vi "FTW-JSON-Object-SetElement-DBL.vi"(0 "JSON Object":refnum<data-value>, 5 "Key":string, 7 "Value":dbl, 11 "error in":errorcluster) -> (4 "JSON Object out":refnum<data-value>, 15 "error out":errorcluster)   [LabVIEW 2014]
uses:
  core/FTW-JSON-Core-Structure.ctl
  error/FTW-ERR-ThrowGenericError.vi
  error/FTW-ERR-ThrowError.vi
  error/FTW-ERR-NoErrorConstant.vi
  error/FTW-ERR-CallChain.vi
  string/FTW-STR-ReplaceWhitespace.vi
panel:
  # "Inputs"
  # "Outputs"
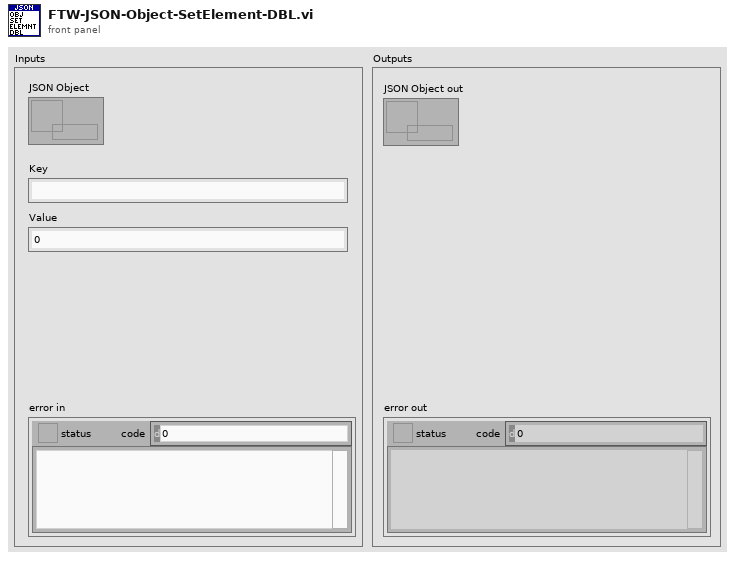
[diagram p1: front panel]
types:
  T1 = typedef "FTW-JSON-Core-Structure.ctl" = cluster{"JSON Object":i64, "Encoding Flags":i64, "Decoding Flags":i64}
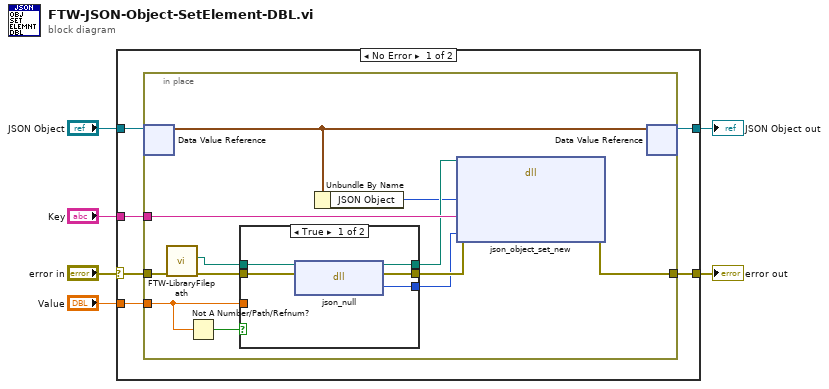
[diagram p0: block diagram]
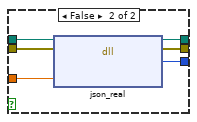
[diagram p2: hidden frame]
diagram:
  n1 = case shown="No Error" "error in" {
    selector: "error in" -> [w12 w37]
    tunnel: [w11 w37] -> w6
    tunnel: [w7 w36] -> w4
    tunnel: "JSON Object" -> [w8 w36]
    tunnel: "Key" -> [w10 _]
    tunnel: "Value" -> [w9 _]
    frame No Error {
      n2 = in-place {
        in-place-border: w12 -> [w24]
        in-place-border: [w23] -> w11
        in-place-border: w10 -> [w22]
        in-place-border: w9 -> [w16]
        n3 = in-place-dvr #1(w8) -> (w14:T1)  [unwired: 1 out]
        n4 = call "FTW-LibraryFilepath.vi"("error in"=w24) -> ("error out"=w19:errorcluster, "Library Filepath"=w21:path)  [unwired: 8 in, 1 out]
        n5 = Not A Number/Path/Refnum?(number/path/refnum=w16) -> (NaN/Path/Refnum?=w15:bool)
        n6 = case shown="True" w15 {
          tunnel: w21 -> [w29 w35]
          tunnel: [w28 w34] -> w20
          tunnel: w19 -> [w27 w33]
          tunnel: [w26 w32] -> w18
          tunnel: w16 -> [_ w31]
          tunnel: [w25 w30] -> w17
          frame True {
            n7 = dll-call lib="?" fn="json_null"(path in=w29, error in=w27) -> (path out=w28:path, error out=w26:errorcluster, "null Value"=w25:i64)  [unwired: 1 in]
          }
          frame False {
            n8 = dll-call lib="?" fn="json_real"(path in=w35, error in=w33, "Double Value"=w31) -> (path out=w34:path, error out=w32:errorcluster, "New Double Value"=w30:i64)  [unwired: 2 in]
          }
        }
        n9 = Unbundle By Name(w14) -> ("JSON Object"=w13:i64)
        n10 = dll-call lib="?" fn="json_object_set_new"(path in=w20, error in=w18, "JSON Object Pointer"=w13, "Key"=w22, "New JSON Object"=w17) -> (error out=w23:errorcluster)  [unwired: 5 in, 1 out]
        n11 = in-place-dvr #1(w14) -> (w7:refnum<data-value>)  [unwired: 1 out]
      }
    }
    frame Error {
    }
  }
  "error out" <- w6
  "JSON Object out" <- w4
